vi "Sort Sync Mask with Schedules.vi"(8 "error in (no error)":errorcluster, 11 "Tamer in":refnum<class "Tamer.lvclass">=refnum) -> (0 "error out":errorcluster, 3 "Tamer out":refnum<class "Tamer.lvclass">)   [LabVIEW 2020, in "CIRCUS_uServices.lvlib" / "Holy Trinity.lvlib" / "Tamer.lvlib" / "Tamer.lvclass"]
uses:
  Tamer.lvclass
  1905bdb5-c98e-4c40-a05c-e821c862ae70.vi
  TALOS/TALOS_PPL.lvlibp
  Run Utilities/Schedule/Schedule.lvclass
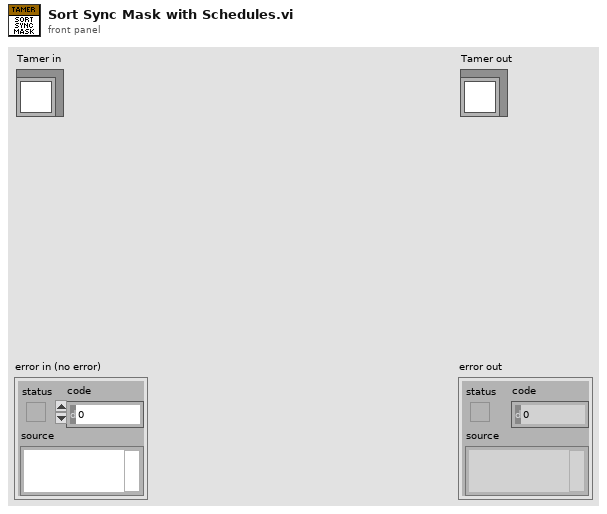
[diagram p1: front panel]
types:
  T1 = typedef "CIRCUS_uServices.lvlib/Run Utilities.lvlib/Synchronize FPGA Cluster.ctl" = cluster{"Status":bool, "FPGA Name":string}
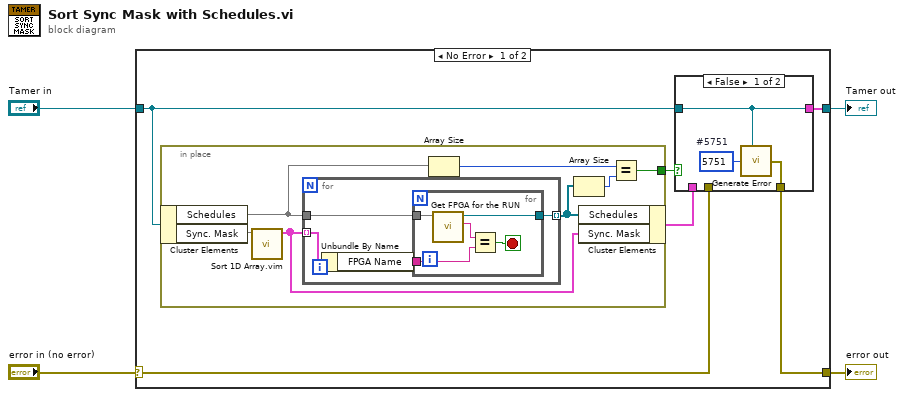
[diagram p0: block diagram]
diagram:
  n1 = case shown="No Error" "error in (no error)" {
    selector: "error in (no error)" -> [w5 w33]
    tunnel: [w6 w33] -> w3
    tunnel: [w8 w32] -> w1
    tunnel: "Tamer in" -> [w7 w32]
    frame No Error {
      n2 = in-place {
        in-place-border: [w17] -> w10
        n3 = in-place-cluster #1(w7) -> ("Schedules"=w21, "Sync. Mask"=w16)
        n4 = call "Sort 1D Array.vim"("unsorted array"=w16) -> ("sorted array"=w22:T1[])  [unwired: 10 in]
        n5 = for {
          tunnel: w21 -> [w25]
          tunnel: w22 -> [w26] mode=indexing
          tunnel: [w23] -> w18 mode=indexing
          n6 = Unbundle By Name(w26) -> ("FPGA Name"=w24:string)
          n7 = for {
            tunnel: w25 -> [w31]
            tunnel: w24 -> [w29]
            tunnel: [w27] -> w23
            stop <- w28 stop-if-true
            n8 = call-dynamic "Get FPGA for the RUN.vi"("Schedule in"=w31) -> ("FPGA Name"=w30:string, "Schedule out"=w27:refnum<class "Schedule.lvclass">)  [unwired: 8 in, 1 out]
            n9 = Equal?(x=w30, y=w29) -> (x = y?=w28:bool)
          }
        }
        n10 = Array Size(array=w21) -> (size(s)=w20:i32)
        n11 = Array Size(array=w18) -> (size(s)=w19:i32)
        n12 = in-place-cluster #1("Schedules"=w18, "Sync. Mask"=w22) -> (w9:cluster{})
        n13 = Equal?(x=w20, y=w19) -> (x = y?=w17:bool)
      }
      n14 = case shown="False" w10 {
        tunnel: w9 -> [_ w15]
        tunnel: [w13 w15] -> w8
        tunnel: w7 -> [w13 _]
        tunnel: [w12 w14] -> w6
        tunnel: w5 -> [_ w14]
        frame False {
          w11 = 5751  # #5751
          n15 = call "Generate Error.vi"("Class"=w13, "Error Code"=w11) -> ("error out"=w12:errorcluster)  [unwired: 5 in]
        }
        frame True {
        }
      }
    }
    frame Error {
    }
  }
  "error out" <- w3
  "Tamer out" <- w1
